vi "Spartan HTTP Log Access Error.vi"(7 "env":T1, 8 "error in (no error)":errorcluster, 10 "reason":string, 11 "absolute path":string) -> (0 "error out":errorcluster)   [LabVIEW 2011]
uses:
  ITK EXT/utils/keyedarr.llb/Keyed Array.ctl
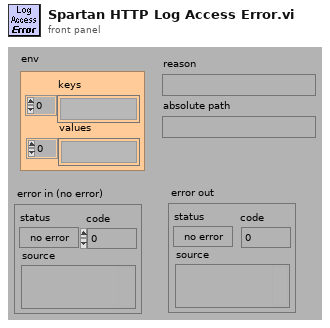
[diagram p1: front panel]
types:
  T1 = typedef "Keyed Array.ctl" = cluster{"keys":string[], "values":string[]}
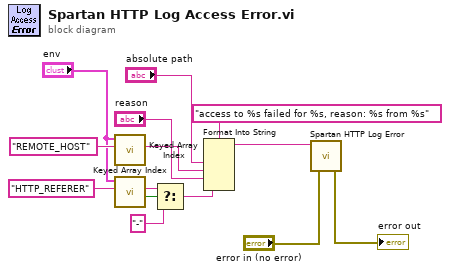
[diagram p0: block diagram]
diagram:
  n1 = call "Keyed Array Index.vi"("key"="REMOTE_HOST", "array in"="env") -> ("value"=w10:string)  [unwired: 2 in, 3 out]
  n2 = call "Keyed Array Index.vi"("key"="HTTP_REFERER", "array in"="env") -> ("valid key"=w3:bool, "value"=w2:string)  [unwired: 2 in, 2 out]
  n3 = Select(t=w2, s=w3, f="-") -> (s? t:f=w4:string)
  n4 = Format Into String(format string="access to %s failed for %s, reason: %s from %s", "absolute path", w10, "reason", w4) -> (resulting string=w8:string)  [unwired: 2 in, 1 out]
  n5 = call "Spartan HTTP Log Error.vi"("error in (no error)"="error in (no error)", "message"=w8) -> ("error out"=→"error out":errorcluster)  [unwired: 1 in, 4 out]
